vi "Temperature Check.vi"(8 "에러 입력 (에러 없음)":errorcluster caption="에러 입력(에러 없음)", 9 "고온":dbl, 10 "저온":dbl, 11 "현재 온도":dbl) -> (0 "에러 출력":errorcluster, 1 "온도 경고?":bool, 2 "온도 경고":string)   [LabVIEW 2010]
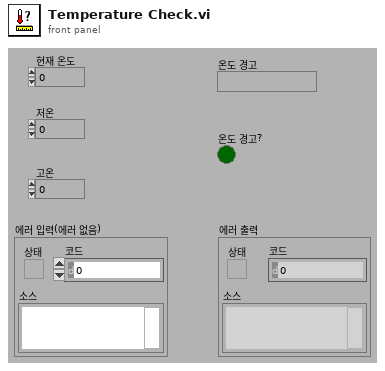
[diagram p1: front panel]
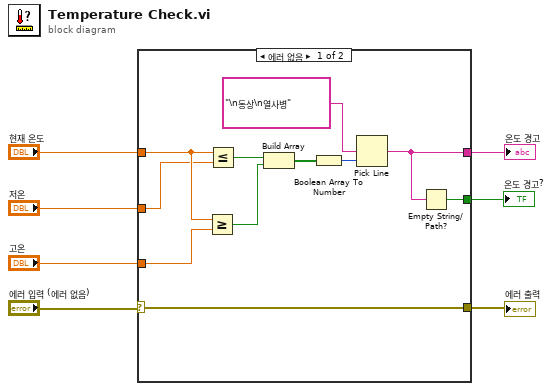
[diagram p0: block diagram]
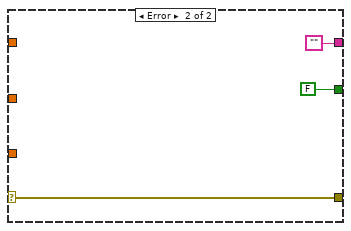
[diagram p2: hidden frame]
diagram:
  n1 = case shown="에러 없음" "에러 입력 (에러 없음)" {
    selector: "에러 입력 (에러 없음)" -> [w8 w21]
    tunnel: "현재 온도" -> [w13 _]
    tunnel: "저온" -> [w12 _]
    tunnel: "고온" -> [w11 _]
    tunnel: [w10 ""] -> w4
    tunnel: [w9 FALSE] -> w3
    tunnel: [w8 w21] -> w1
    frame No Error {
      n2 = Greater Or Equal?(x=w13, y=w11) -> (x >= y?=w15:bool)
      n3 = Less Or Equal?(x=w13, y=w12) -> (x <= y?=w14:bool)
      n4 = Build Array(w14, w15) -> (w16:bool[])
      n5 = Boolean Array To Number(Boolean array=w16) -> (number=w17:u32)
      n6 = Pick Line(multi-line string="\n동상\n열사병", line index=w17) -> (output string=w10:string)  [unwired: 1 out]
      n7 = Empty String/Path?(string/path=w10) -> (empty?=w9:bool)
    }
    frame Error {
    }
  }
  "온도 경고" <- w4
  "온도 경고?" <- w3
  "에러 출력" <- w1
